vi "Initialize Cfg Datw.vi"(6 "Qo2":sgl[](array[numeric])=[1.0, 0.75, 0.5, 0.25] caption="O2 flows", 7 "numObs":u16=20 caption="Number of Points\nto Collect", 8 "error in":errorcluster, 10 "waits":T1={"Zero"=12.0, "Purge"=10.0, "O3 Stability"=0.0, "Laser Stability"=12.0} caption="Wait Times (s)", 11 "Calibration UI in":refnum<class "Calibration UI.lvclass">) -> (0 "error out":errorcluster, 1 "Stored Data":refnum<data-value>, 2 "Cfg Array":refnum<class "Data.lvclass">[](array[class]), 3 "Calibration UI out":refnum<class "Calibration UI.lvclass">)   [LabVIEW 2015, in "Calibration UI.lvclass"]
uses:
  Calibration UI.lvclass
  Reusable/Data/Data.lvclass
  Calibration/State data/State Data.lvclass
  Reusable/Data/Array Data/Single 1-D/Single_Array.lvclass
  Reusable/Data/Double/Double.lvclass
  Reusable/Data/U16/U16.lvclass
  Calibration/Associated data/Associated Data.lvclass
  Calibration/Data DVR/cPAS Data DVR.lvclass
  Reusable/Data/Boolean/Boolean Data.lvclass
  Controls/Flags.ctl
  Calibration UI.lvclass/Calibration UI.ctl
  Calibration/Data DVR/cPAS Data DVR.lvclass/cPAS Data DVR.ctl
  Calibration/Associated data/Associated Data.lvclass/Associated Data.ctl
  Reusable/Data/Boolean/Boolean Data.lvclass/Boolean Data.ctl
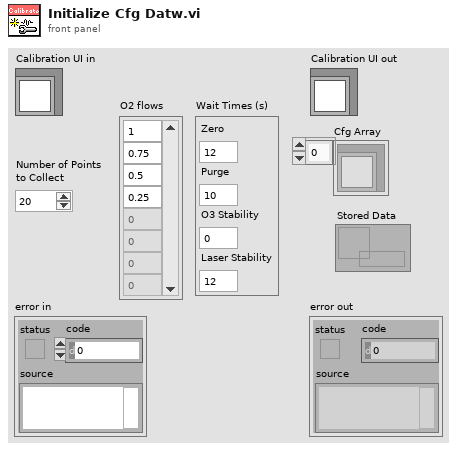
[diagram p1: front panel]
types:
  T1 = cluster{"Zero":dbl, "Purge":dbl, "O3 Stability":dbl, "Laser Stability":dbl}
  T2 = typedef "Flags.ctl" = enum8{"Autospeaker", "Link cycles", "Autofilter", "O3 Cal", "Filter Position"}
  T3 = cluster{"Stored State":refnum<class "State Data.lvclass">[], "pointer to data":i32}
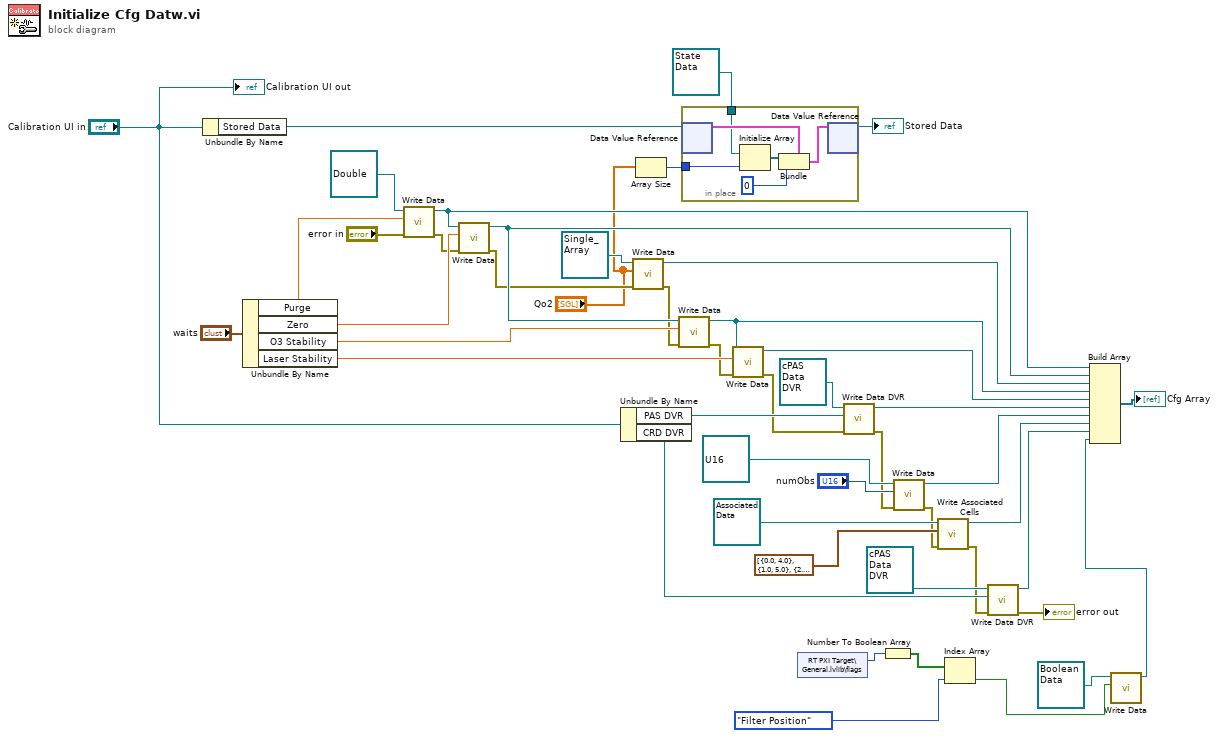
[diagram p0: block diagram]
diagram:
  n1 = Unbundle By Name("Calibration UI in") -> ("Stored Data"=w8:refnum<data-value>)
  n2 = Unbundle By Name("waits") -> ("Purge"=w39:dbl, "Zero"=w40:dbl, "O3 Stability"=w41:dbl, "Laser Stability"=w42:dbl)
  n3 = call "Write Data.vi"("error in (no error)"="error in", "Data"=w39, "Double in"=refnum<class "Double.lvclass"> refnum ("Base Data Class.lvlib:Double.lvclass")) -> ("error out"=w21:errorcluster, "Double out"=w28:refnum<class "Double.lvclass">)  [unwired: 7 in]
  n4 = call "Write Data.vi"("error in (no error)"=w21, "Data"=w40, "Double in"=w28) -> ("error out"=w20:errorcluster, "Double out"=w37:refnum<class "Double.lvclass">)  [unwired: 7 in]
  n5 = Unbundle By Name("Calibration UI in") -> ("PAS DVR"=w24:refnum<data-value>, "CRD DVR"=w23:refnum<data-value>)
  n6 = call "Write Data.vi"("error in (no error)"=w20, "Data"="Qo2", "Single_Array in"=refnum<class "Single_Array.lvclass"> refnum ("Base Data Class.lvlib:Single_Array.lvclass")) -> ("error out"=w19:errorcluster, "Single_Array out"=w29:refnum<class "Single_Array.lvclass">)  [unwired: 7 in]
  n7 = Array Size(array="Qo2") -> (size(s)=w12:i32)
  n8 = call "Write Data.vi"("error in (no error)"=w19, "Data"=w41, "Double in"=w37) -> ("error out"=w18:errorcluster, "Double out"=w43:refnum<class "Double.lvclass">)  [unwired: 7 in]
  n9 = in-place {
    in-place-border: w12 -> [w49]
    in-place-border: refnum<class "State Data.lvclass"> refnum ("State Data") -> [w48]
    n10 = in-place-dvr #1(w8) -> (w51:T3)  [unwired: 1 out]
    n11 = Initialize Array(w48, w49) -> (w53:refnum<class "State Data.lvclass">[])
    n12 = Bundle(cluster=w51, "Stored State"=w53, "pointer to data"=0) -> (w50:T3)
    n13 = in-place-dvr #1(w50) -> (→"Stored Data":refnum<data-value>)  [unwired: 1 out]
  }
  n14 = call "Write Data.vi"("error in (no error)"=w18, "Data"=w42, "Double in"=w43) -> ("error out"=w17:errorcluster, "Double out"=w38:refnum<class "Double.lvclass">)  [unwired: 7 in]
  n15 = shared-variable "RT PXI Target\\General.lvlib\\flags"() -> (w6:u8)  [unwired: 1 in, 1 out]
  n16 = call "Write Data DVR.vi"("error in (no error)"=w17, "Data DVR"=w24, "cPAS Data DVR in"=refnum<class "cPAS Data DVR.lvclass"> refnum ("cPAS Data DVR.lvclass")) -> ("error out"=w16:errorcluster, "cPAS Data DVR out"=w31:refnum<class "cPAS Data DVR.lvclass">)  [unwired: 7 in]
  n17 = Number To Boolean Array(number=w6) -> (Boolean array=w5:bool[])
  n18 = call "Write Data.vi"("error in"=w16, "Data"="numObs", "U16 in"=refnum<class "U16.lvclass"> refnum ("Base Data Class.lvlib:U16")) -> ("error out"=w15:errorcluster, "U16 out"=w34:refnum<class "U16.lvclass">)  [unwired: 7 in]
  n19 = call "Write Associated Cells.vi"("error in (no error)"=w15, "Associated Cells"=cluster{"PAS":dbl, "CRD":dbl}[] [{"PAS"=0.0, "CRD"=4.0}, {"PAS"=1.0, "CRD"=5.0}, {"PAS"=2.0, "CRD"=4.0}, {"PAS"=3.0, "CRD"=3.0}, {"PAS"=4.0, "CRD"=3.0}], "Associated Data in"=refnum<class "Associated Data.lvclass"> refnum ("Associated Data.lvclass")) -> ("error out"=w14:errorcluster, "Associated Data out"=w35:refnum<class "Associated Data.lvclass">)  [unwired: 7 in]
  n20 = Index Array(array=w5, index=Flags."Filter Position" ("Flags")) -> (element=w3:bool)
  n21 = call "Write Data DVR.vi"("error in (no error)"=w14, "Data DVR"=w23, "cPAS Data DVR in"=refnum<class "cPAS Data DVR.lvclass"> refnum ("cPAS Data DVR.lvclass")) -> ("error out"=→"error out":errorcluster, "cPAS Data DVR out"=w36:refnum<class "cPAS Data DVR.lvclass">)  [unwired: 7 in]
  n22 = call "Write Data.vi"("Data"=w3, "Boolean Data in"=refnum<class "Boolean Data.lvclass"> refnum ("Boolean Data.lvclass")) -> ("Boolean Data out"=w2:refnum<class "Boolean Data.lvclass">)  [unwired: 8 in, 1 out]
  n23 = Build Array(w28, w37, w29, w43, w38, w31, w34, w35, w36, w2) -> (→"Cfg Array":refnum<class "Data.lvclass">[])
  "Calibration UI out" <- "Calibration UI in"
